vi "SBML_Rules.vi"(8 "error in (no error)":errorcluster, 11 "Input SBML File":string) -> (0 "error out":errorcluster, 2 "Rules":string[][](table), 3 "RulesCnt":i32)   [LabVIEW 2014]
doc: "This VI extract the information of species present in SBML file. It takes the complete SBML file as input, and outputs: \nSp_Cnt --> How many species are there\nS_Id_Arr --> Array of species\nSp_Name --> Array containing the name of species\nSp_Init_Amnt --> Array containing the initial amount of species\n\nDesigned by HB\nhaba@dtu.dk"
panel:
  out "RuleMath":string[](array[string])
  out "RuleVar":string[](array[string])
  out "RuleMetaID":string[](array[string])
  out "RuleType":string[](array[string])
  out "List of Rules":string
  # "Names"
  # "Initial Amount"
  # "ID"
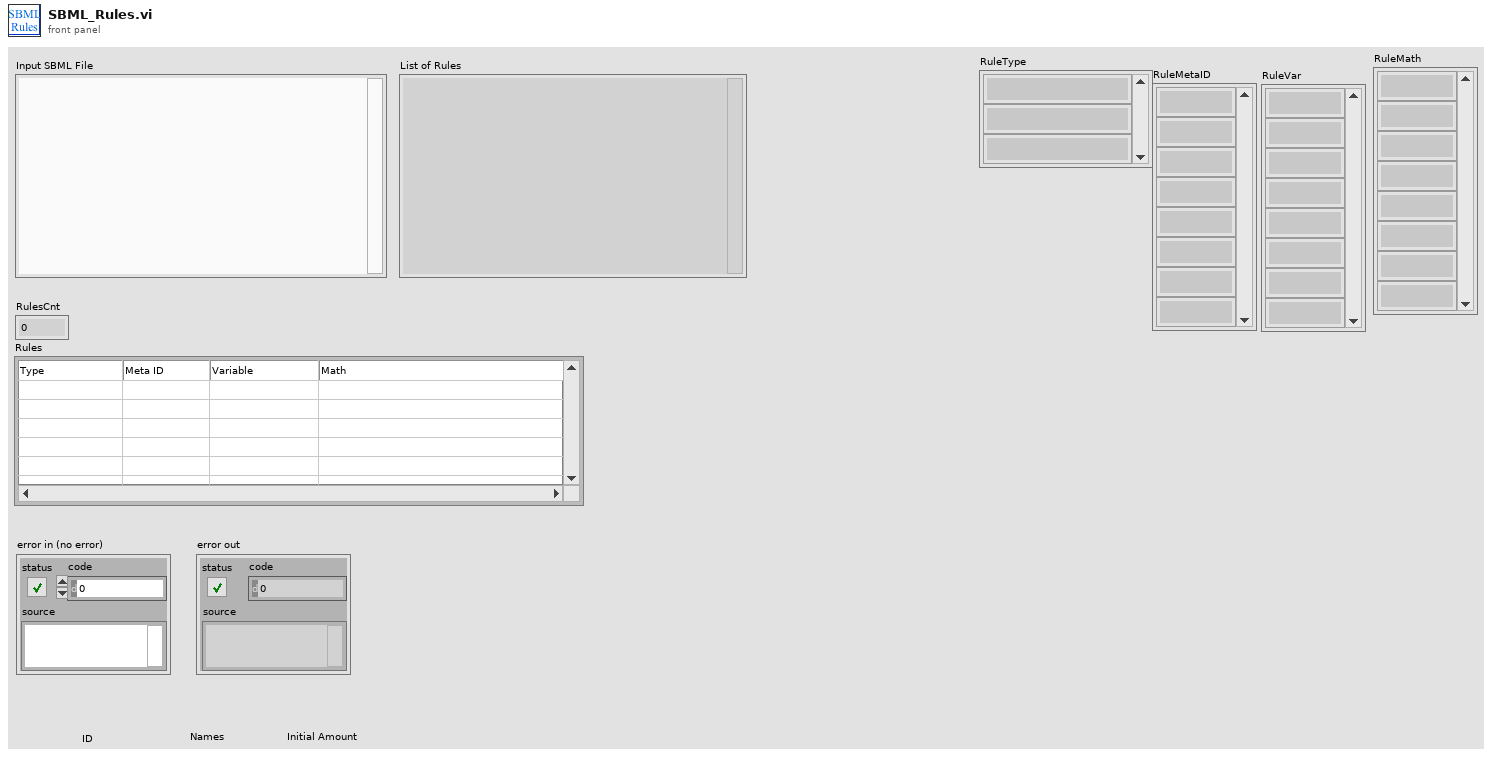
[diagram p1: front panel]
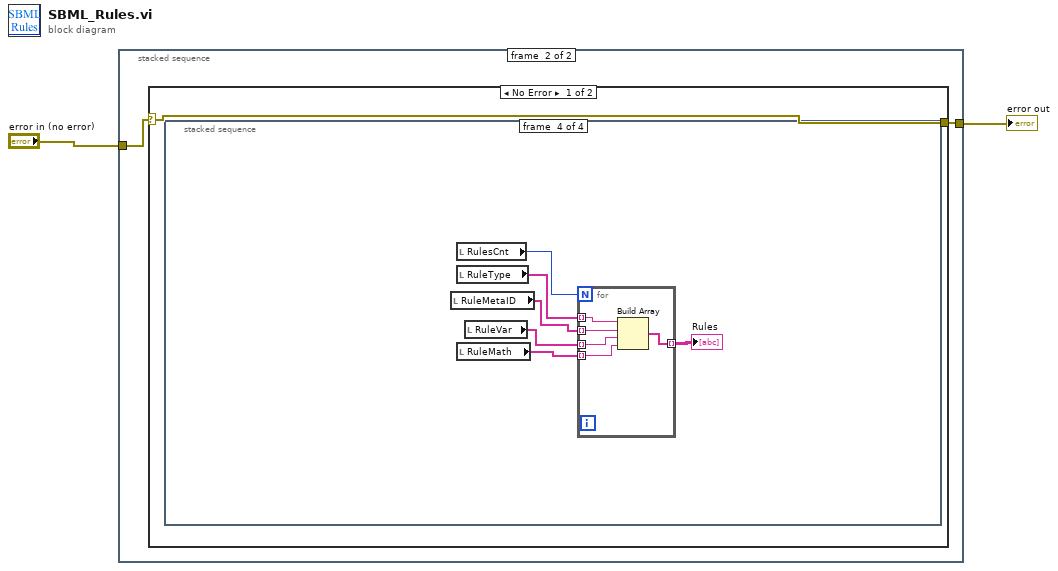
[diagram p0: block diagram]
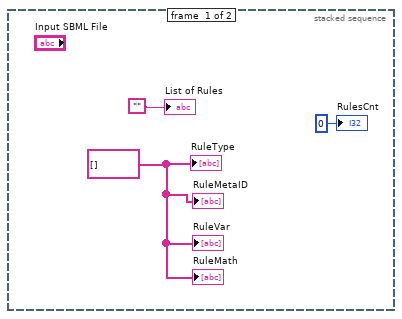
[diagram p2: hidden frame]
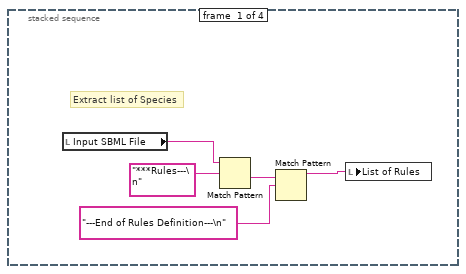
[diagram p3: hidden frame]
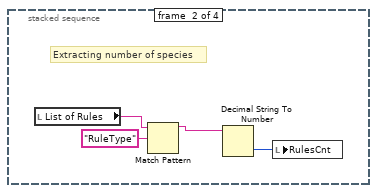
[diagram p4: hidden frame]
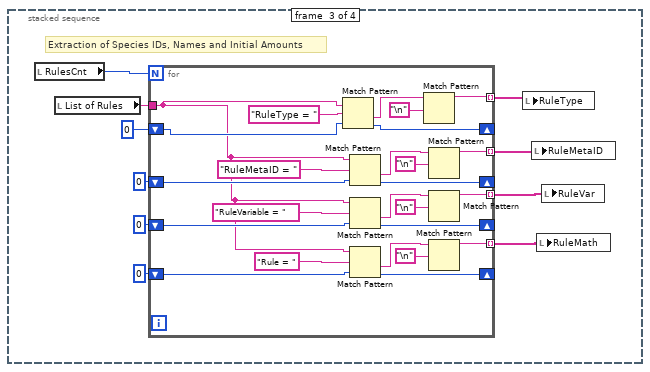
[diagram p5: hidden frame]
diagram:
  n1 = stacked-sequence {
    tunnel: "error in (no error)" -> [_ w6]
    tunnel: [_ w7] -> w1
    frame #0 {
      w3 = string[] [] ("Sp_Id_Arr")
      "List of Rules" <- "" ("Full SBML File")
      "RulesCnt" <- 0 ("Sp_cnt")
      "RuleType" <- w3
      "RuleMetaID" <- w3
      "RuleVar" <- w3
      "RuleMath" <- w3
    }
    frame #1 {
      n2 = case shown="No Error" w6 {
        selector: w6 -> [w8 w64]
        tunnel: [w8 w64] -> w7
        frame No Error {
          n3 = stacked-sequence {
            frame #0 {
              # "Extract list of Species"
              n4 = local read "Input SBML File"() -> (w10:string)
              n5 = Match Pattern(string=w10, regular expression="***Rules---\n") -> (after substring=w12:string)  [unwired: 1 in, 3 out]
              n6 = Match Pattern(string=w12, regular expression="---End of Rules Definition---\n") -> (before substring=w9:string)  [unwired: 1 in, 3 out]
              n7 = local write "List of Rules"(w9) -> ()
            }
            frame #1 {
              # "Extracting number of species"
              n8 = local read "List of Rules"() -> (w14:string)
              n9 = Match Pattern(string=w14, regular expression="RuleType") -> (before substring=w15:string)  [unwired: 1 in, 3 out]
              n10 = Decimal String To Number(string=w15) -> (number=w17:i32)  [unwired: 2 in, 1 out]
              n11 = local write "RulesCnt"(w17) -> ()
            }
            frame #2 {
              # "Extraction of Species IDs, Names and Initial Amounts"
              n12 = local read "RulesCnt"() -> (w25:i32)
              n13 = local read "List of Rules"() -> (w26:string)
              n14 = for {
                N: w25 -> [_]
                tunnel: w26 -> [w28]
                shift-right: [w41] -> _
                shift-left: 0 ("offset past match") -> [w42]
                tunnel: [w49] -> w24 mode=indexing
                shift-right: [w46] -> _
                shift-left: 0 ("offset past match") -> [w47]
                tunnel: [w48] -> w23 mode=indexing
                shift-right: [w37] -> _
                shift-left: 0 ("offset past match") -> [w36]
                tunnel: [w35] -> w20 mode=indexing
                shift-right: [w32] -> _
                shift-left: 0 ("offset past match") -> [w33]
                tunnel: [w34] -> w19 mode=indexing
                n15 = Match Pattern(string=w28, regular expression="RuleType = ", offset (0)=w42) -> (after substring=w50:string, offset past match=w41:i32)  [unwired: 2 out]
                n16 = Match Pattern(string=w28, regular expression="RuleMetaID = ", offset (0)=w47) -> (after substring=w43:string, offset past match=w46:i32)  [unwired: 2 out]
                n17 = Match Pattern(string=w28, regular expression="RuleVariable = ", offset (0)=w36) -> (after substring=w40:string, offset past match=w37:i32)  [unwired: 2 out]
                n18 = Match Pattern(string=w28, regular expression="Rule = ", offset (0)=w33) -> (after substring=w29:string, offset past match=w32:i32)  [unwired: 2 out]
                n19 = Match Pattern(string=w50, regular expression="\n") -> (before substring=w49:string)  [unwired: 1 in, 3 out]
                n20 = Match Pattern(string=w43, regular expression="\n") -> (before substring=w48:string)  [unwired: 1 in, 3 out]
                n21 = Match Pattern(string=w40, regular expression="\n") -> (before substring=w35:string)  [unwired: 1 in, 3 out]
                n22 = Match Pattern(string=w29, regular expression="\n") -> (before substring=w34:string)  [unwired: 1 in, 3 out]
              }
              n23 = local write "RuleType"(w24) -> ()
              n24 = local write "RuleMetaID"(w23) -> ()
              n25 = local write "RuleMath"(w19) -> ()
              n26 = local write "RuleVar"(w20) -> ()
            }
            frame #3 {
              n27 = local read "RuleMetaID"() -> (w55:string[])
              n28 = local read "RulesCnt"() -> (w56:i32)
              n29 = local read "RuleType"() -> (w54:string[])
              n30 = local read "RuleMath"() -> (w53:string[])
              n31 = local read "RuleVar"() -> (w57:string[])
              n32 = for {
                N: w56 -> [_]
                tunnel: w54 -> [w63] mode=indexing
                tunnel: w55 -> [w62] mode=indexing
                tunnel: [w61] -> w58 mode=indexing
                tunnel: w57 -> [w60] mode=indexing
                tunnel: w53 -> [w59] mode=indexing
                n33 = Build Array(w63, w62, w60, w59) -> (w61:string[])
              }
              "Rules" <- w58
            }
          }
        }
        frame Error {
        }
      }
    }
  }
  "error out" <- w1
